vi "Monitor DNA length.vi"(5 "OK Button":bool caption="Reset BM", 6 "initial parameters":dbl[](array[numeric])=[15.0, 2.0, 15.0, 2.0, 100.0, 127.0], 7 "Input Image":T1(plugin-control)) -> (2 "Results":dbl[](array[numeric]))   [LabVIEW 2014]
uses:
  <vilib>/gmath/NI_Gmath.lvlib
  <vilib>/Analysis/NI_AALBase.lvlib
  <vilib>/Math Plots/3D Math Plots/3D Scatter/3D Scatter Datatype/3D Scatter Datatype.lvclass
  <vilib>/Analysis/baseanly.llb/Mean (DBL).vi
  <vilib>/Analysis/1siggen.llb/Ramp Pattern by Samples.vi
  <vilib>/gmath/NumericalOptimization/Nonlinear Curve Fit LM.vi
  <vilib>/Math Plots/3D Math Plots/3D Scatter/3D Scatter Datatype/Public/Plot Helper (Vector).vi
  <vilib>/Math Plots/3D Math Plots/3D Scatter/3D Scatter Datatype/Public/Plot Helper (Matrix).vi
  <vilib>/Math Plots/3D Math Plots/3D Scatter/3D Scatter XCtrl/3D Scatter.xctl
panel:
  out "BMx array(pixel)":dbl[](array[numeric])
  in  "Tab Control":enum32{"DNA", "Image", "Results"}(tab)
  out "3D Scatter":refnum<class "3D Plot Datatype.lvclass">[](xcontrol)
  out "BMy":dbl(graph)
  out "BMx":dbl(graph)
  out "BMy":dbl[](array[numeric])
  out "y position appended array":dbl[](array[numeric])
  out "image size(pixel)":i32
  out "updated BMy (nm)":dbl
  out "updated BMx (nm)":dbl
  out "cf (nm/pixel)":dbl
  out "BMx":dbl[](array[numeric])
  out "x position appended array":dbl[](array[numeric])
  in  "BM window size":i32=10
  out "xy ratio":dbl
  out "updated BMy (pixel)":dbl format="%0.2f"
  out "updated BMx (pixel)":dbl format="%0.2f"
  out "y position":dbl
  out "x position":dbl
  in  "stop":bool
  out "error out":errorcluster
  out "best fit parameters":dbl[](array[numeric])
  out "Parameter Names":string[](array[string])=["Xposition", "Xwidth", "Yposition", "Ywidth", "Amplitude", "Offset"]
  in  "Image Pixels (U8) 2":u8[][](array[numeric])=[[60, 70, 80, 50, 30], [100, 160, 150, 110, 30], [100, 170, 200, 150, 70], [100, 140, 150, 120, 60], [80, 70, 80, 60, 20]]
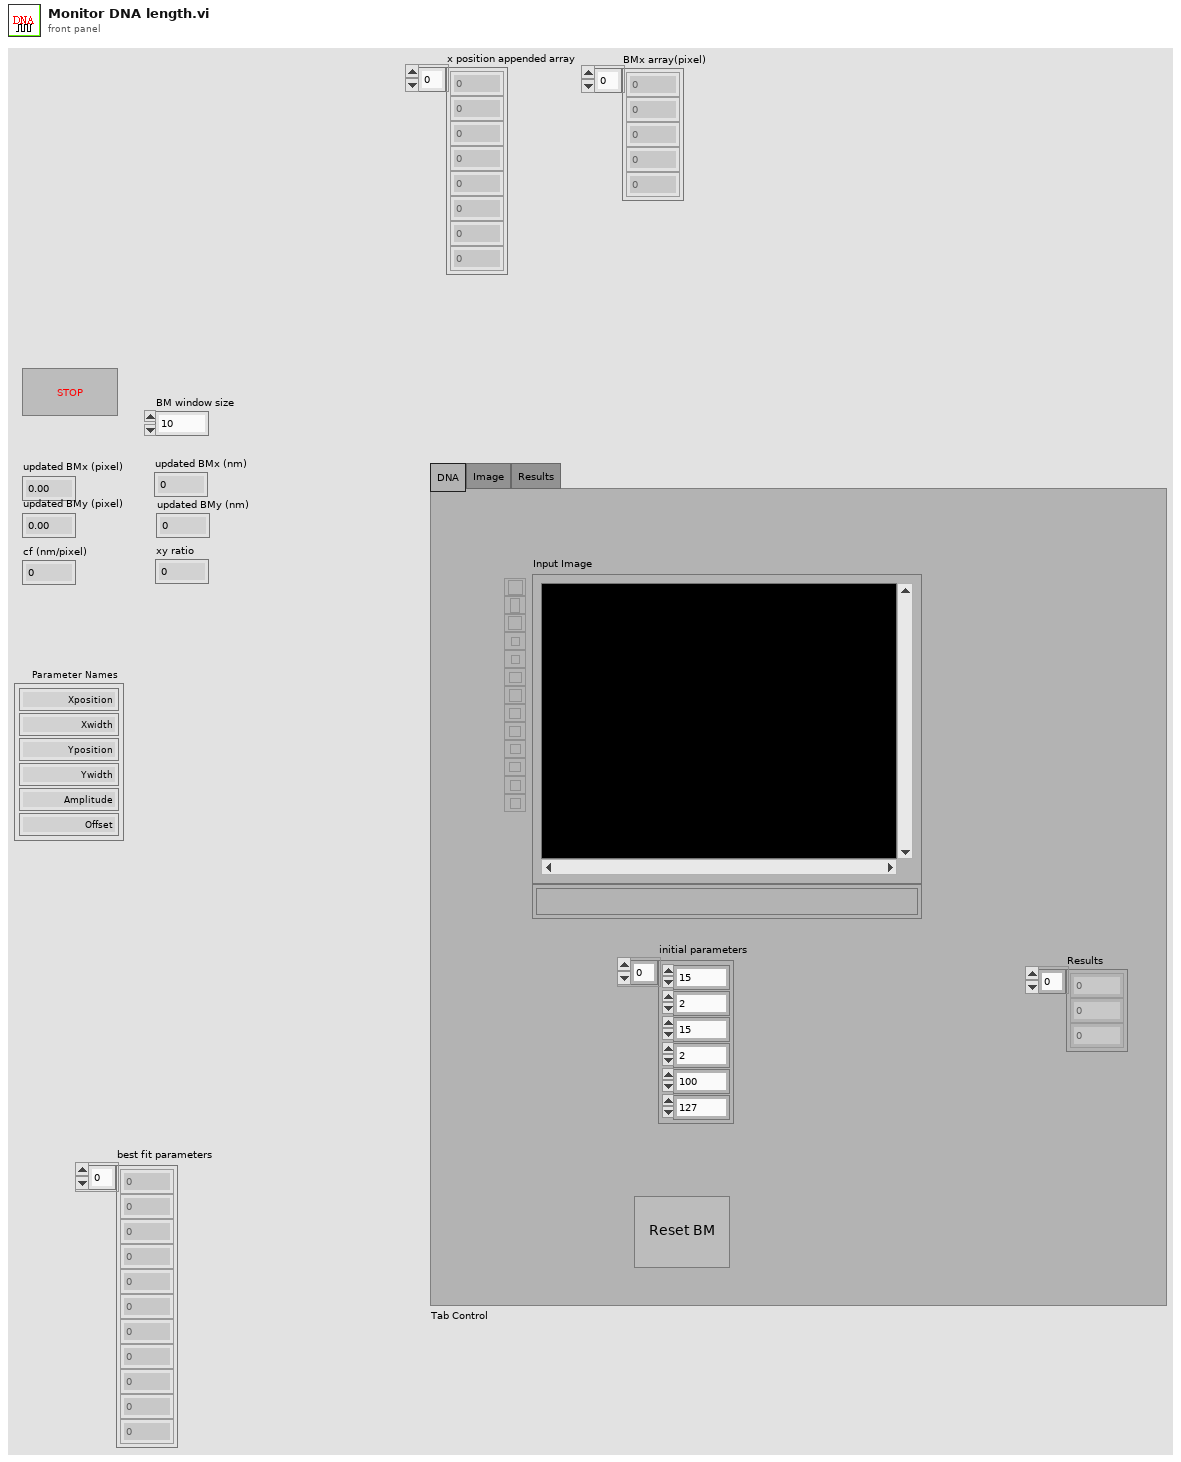
[diagram p1: front panel]
types:
  T1 = typedef "IMAQ Image.ctl" = refnum<image>
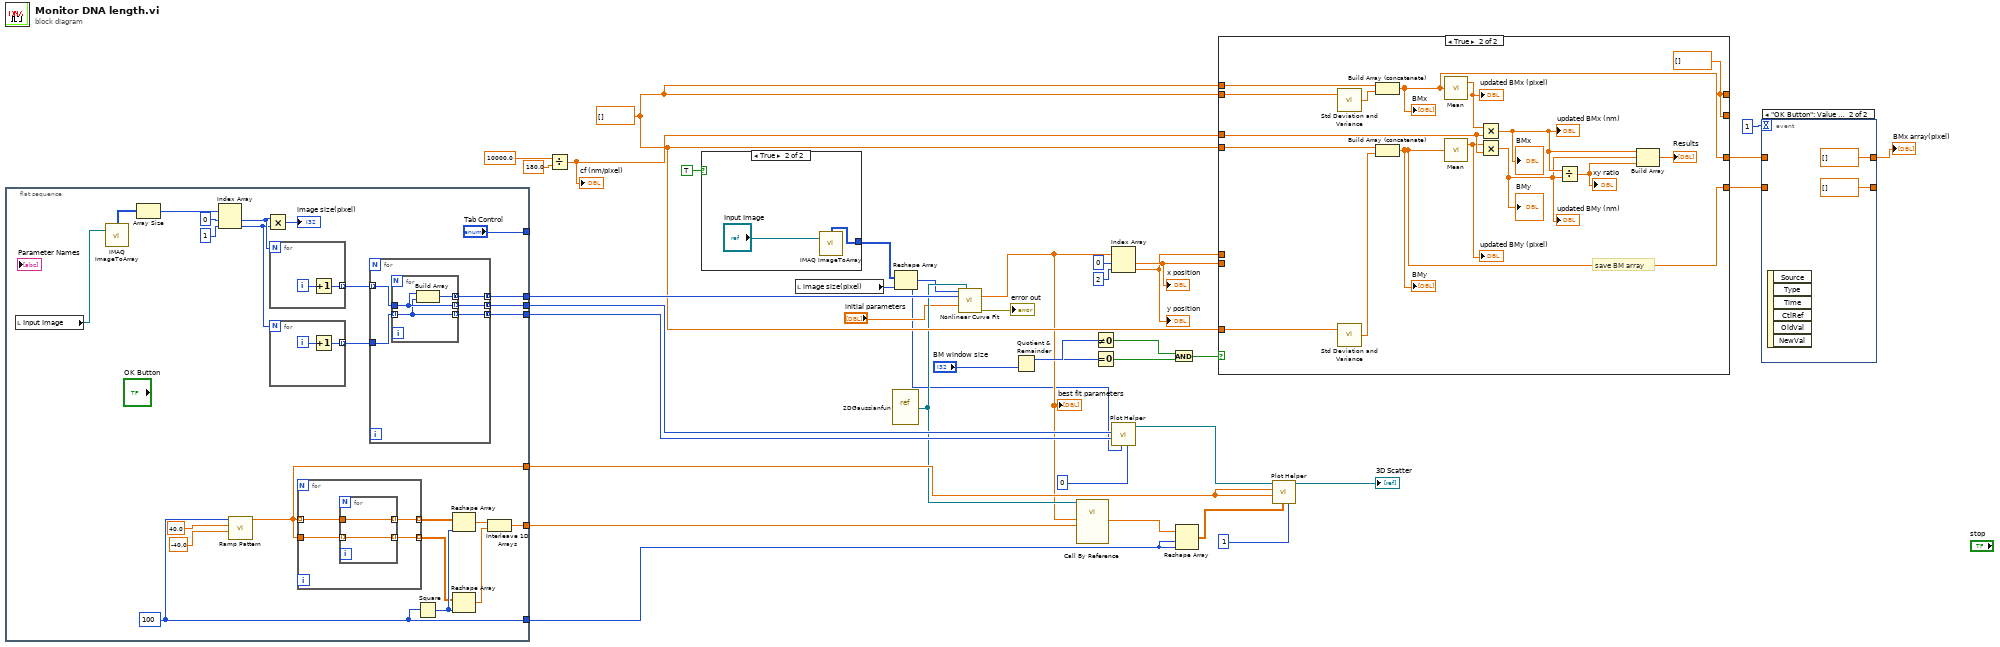
[diagram p0: block diagram]
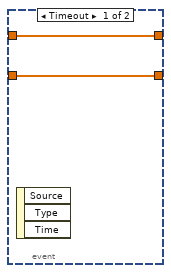
[diagram p2: hidden frame]
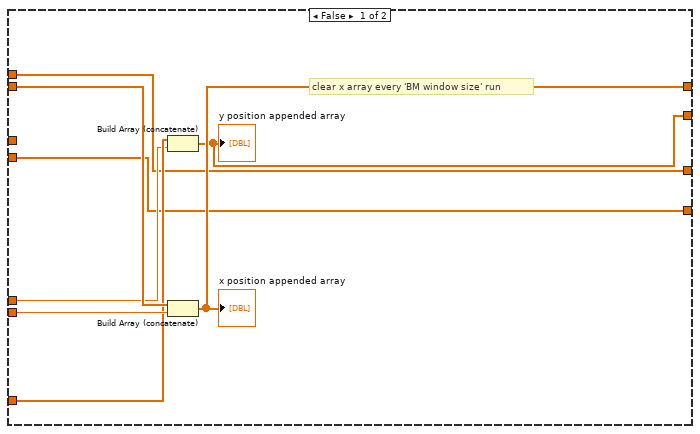
[diagram p3: hidden frame]
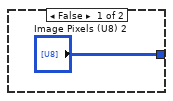
[diagram p4: hidden frame]
diagram:
  w32 = dbl[] []
  n1 = flat-sequence {
    tunnel: [w57] -> w41
    tunnel: [w56] -> w40
    tunnel: [w55] -> w39
    tunnel: [w51] -> w38
    tunnel: [w50] -> w37
    tunnel: [w44] -> w36
    tunnel: ["Tab Control"] -> _
    frame #0 {
      w50 = 100 ("samples")
      n2 = local read "Input Image"() -> (w42:T1)
      n3 = call "IMAQ ImageToArray"("Image"=w42) -> ("Image Pixels (U8)"=w63:u8[][])  [unwired: 3 in, 4 out]
      n4 = Array Size(array=w63) -> (size(s)=w62:i32[])
      n5 = Index Array(array=w62, index #1=0 ("index"), index #2=1 ("index")) -> (element #1=w61:i32, element #2=w60:i32)
      n6 = call-poly <vilib>:"Ramp Pattern.vi"("start"=-40.0, "end"=40.0, "samples"=w50) -> ("Ramp Pattern"=w51:dbl[])  [unwired: 7 in, 1 out]
      n7 = Multiply(x=w61, y=w60) -> (x*y=→"image size(pixel)":i32)
      n8 = for {
        N: w61 -> [_]
        tunnel: [w82] -> w59 mode=indexing
        i -> [w83]
        n9 = Increment(x=w83) -> (x+1=w82:i32)
      }
      n10 = for {
        N: w60 -> [_]
        tunnel: [w80] -> w58 mode=indexing
        i -> [w81]
        n11 = Increment(x=w81) -> (x+1=w80:i32)
      }
      n12 = for {
        tunnel: w51 -> [w69] mode=indexing
        tunnel: w51 -> [w68]
        tunnel: [w67] -> w48 mode=indexing
        tunnel: [w66] -> w47 mode=indexing
        n13 = for {
          tunnel: w69 -> [w71]
          tunnel: w68 -> [w70] mode=indexing
          tunnel: [w71] -> w67 mode=indexing
          tunnel: [w70] -> w66 mode=indexing
        }
      }
      n14 = for {
        tunnel: w59 -> [w76] mode=indexing
        tunnel: w58 -> [w75]
        tunnel: [w74] -> w56 mode=concatenating
        tunnel: [w73] -> w57 mode=concatenating
        tunnel: [w72] -> w55 mode=concatenating
        n15 = for {
          tunnel: w76 -> [w78]
          tunnel: w75 -> [w77] mode=indexing
          tunnel: [w79] -> w74 mode=concatenating
          tunnel: [w78] -> w73 mode=indexing
          tunnel: [w77] -> w72 mode=indexing
          n16 = Build Array(w78, w77) -> (w79:i32[])
        }
      }
      n17 = Square(x=w50) -> (x^2=w49:i32)
      n18 = Reshape Array(w48, w49) -> (w46:dbl[])
      n19 = Reshape Array(w47, w49) -> (w45:dbl[])
      n20 = Interleave 1D Arrays(w46, w45) -> (w44:dbl[])
    }
  }
  n21 = Divide(x=10000.0, y=180.0) -> (x/y=w33:dbl)
  "cf (nm/pixel)" <- w33
  n22 = case shown="True" TRUE {
    tunnel: ["Image Pixels (U8) 2" w86] -> w24
    frame False {
    }
    frame True {
      n23 = call "IMAQ ImageToArray"("Image"="Input Image") -> ("Image Pixels (U8)"=w86:u8[][])  [unwired: 3 in, 4 out]
    }
  }
  n24 = local read "image size(pixel)"() -> (w13:i32)
  n25 = vi-ref "2DGaussianfun.vi"() -> (w31:refnum<vi>)
  n26 = Reshape Array(w24, w13) -> (w12:u8[])
  n27 = call-poly <vilib>:"Nonlinear Curve Fit.vi"("Y"=w12, "f(x,a)"=w31, "X"=w40, "initial parameters"="initial parameters") -> ("best fit parameters"=w21:dbl[], "error out"=→"error out":errorcluster)  [unwired: 6 in, 4 out]
  "best fit parameters" <- w21
  n28 = Quotient & Remainder(y="BM window size") -> (x=w26:i32, x-y*floor(x/y)=w18:i32)  [unwired: 1 out]
  n29 = call-by-ref "?"(reference=w31, "X"=w36, "Coefficients"=w21) -> ("f(X,a)"=w11:dbl[])  [unwired: 3 in, 4 out]
  n30 = Not Equal To 0?(x=w26) -> (x != 0?=w17:bool)
  n31 = Equal To 0?(x=w18) -> (x = 0?=w16:bool)
  n32 = Index Array(array=w21, index #1=0 ("index"), index #2=2 ("index")) -> (element #1=w30:dbl, element #2=w29:dbl)
  "x position" <- w30
  "y position" <- w29
  n33 = call-poly <vilib>:"Plot Helper.vi"("Plot ID"=0, "z vector"=w12, "y vector"=w39, "x vector"=w41) -> ("3D Plot lvclass Array out"=w7:refnum<class "3D Plot Datatype.lvclass">[])  [unwired: 2 in, 5 out]
  n34 = And(x=w17, y=w16) -> (x .and. y?=w15:bool)
  n35 = Reshape Array(w11, w37, w37) -> (w6:dbl[][])
  n36 = case shown="True" w15 {
    tunnel: w32 -> [w94 w110]
    tunnel: w30 -> [w93 _]
    tunnel: [w92 w106] -> w28
    tunnel: w32 -> [w91 w109]
    tunnel: w29 -> [w90 _]
    tunnel: [w89 w106] -> w27
    tunnel: [w87 w102] -> w4
    tunnel: w32 -> [w88 w105]
    tunnel: w33 -> [_ w101]
    tunnel: [w88 w103] -> w5
    tunnel: w32 -> [w87 w100]
    frame False {
      # "clear x array every 'BM window size' run"
      n37 = Build Array (concatenate)(w91, w90) -> (w89:dbl[])
      "y position appended array" <- w89
      n38 = Build Array (concatenate)(w94, w93) -> (w92:dbl[])
      "x position appended array" <- w92
    }
    frame True {
      w106 = dbl[] []
      # "save BM array"
      n39 = call <vilib>:"Std Deviation and Variance.vi"("X"=w110) -> ("standard deviation"=w108:dbl)  [unwired: 1 in, 2 out]
      n40 = call <vilib>:"Std Deviation and Variance.vi"("X"=w109) -> ("standard deviation"=w107:dbl)  [unwired: 1 in, 2 out]
      n41 = Build Array (concatenate)(w105, w108) -> (w103:dbl[])
      "BMx" <- w103
      n42 = Build Array (concatenate)(w100, w107) -> (w102:dbl[])
      "BMy" <- w102
      n43 = call-poly <vilib>:"Mean.vi"("X"=w103) -> ("mean"=w104:dbl)  [unwired: 1 out]
      "updated BMx (pixel)" <- w104
      n44 = call-poly <vilib>:"Mean.vi"("X"=w102) -> ("mean"=w98:dbl)  [unwired: 1 out]
      "updated BMy (pixel)" <- w98
      n45 = Multiply(x=w104, y=w101) -> (x*y=w99:dbl)
      "updated BMx (nm)" <- w99
      "BMx" <- w99
      n46 = Multiply(x=w98, y=w101) -> (x*y=w95:dbl)
      "updated BMy (nm)" <- w95
      "BMy" <- w95
      n47 = Divide(x=w99, y=w95) -> (x/y=w97:dbl)
      "xy ratio" <- w97
      n48 = Build Array(w99, w95, w97) -> (→"Results":dbl[])
    }
  }
  n49 = call-poly <vilib>:"Plot Helper.vi"("Plot ID"=1, "z matrix"=w6, "y vector"=w38, "x vector"=w38, "3D Plot lvclass Array in"=w7) -> ("3D Plot lvclass Array out"=→"3D Scatter":refnum<class "3D Plot Datatype.lvclass">[])  [unwired: 1 in, 5 out]
  n50 = event shown="[1] \"OK Button\": Value Change" {
    selector: _ -> [_ _]
    dyn-events: _ -> [_ _]
    timeout: 1 -> [_ _]
    tunnel: w5 -> [w112 _]
    tunnel: [w112 dbl[] []] -> w2
    tunnel: w4 -> [w111 _]
    tunnel: [w111 dbl[] []] -> w3
    event Timeout {
      n51 = event-data() -> ()  [unwired: 1 in, 3 out]
    }
    event "OK Button": Value Change {
      n52 = event-data() -> ()  [unwired: 1 in, 6 out]
    }
  }
  "BMx array(pixel)" <- w2
